vi "Test DIO.vi"() -> ()   [LabVIEW 2012]
uses:
  <vilib>/DAQmx/write.llb/DAQmx Write (Digital 2D Bool NChan 1Samp NLine).vi
  <vilib>/DAQmx/read.llb/DAQmx Read (Digital 2D Bool NChan 1Samp NLine).vi
  <vilib>/DAQmx/create/channels.llb/DAQmx Create Channel (DO-Digital Output).vi
  <vilib>/DAQmx/miscellaneous.llb/DAQmx Fill In Error Info.vi
panel:
  out "data read":bool[][](array[boolean])
  in  "data":bool[][](array[boolean])
  out "number of samples written per channel":u32
  in  "stop":bool
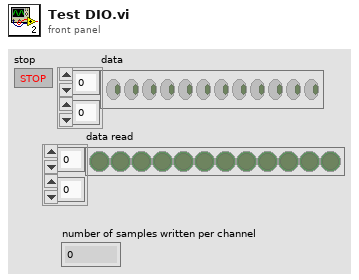
[diagram p1: front panel]
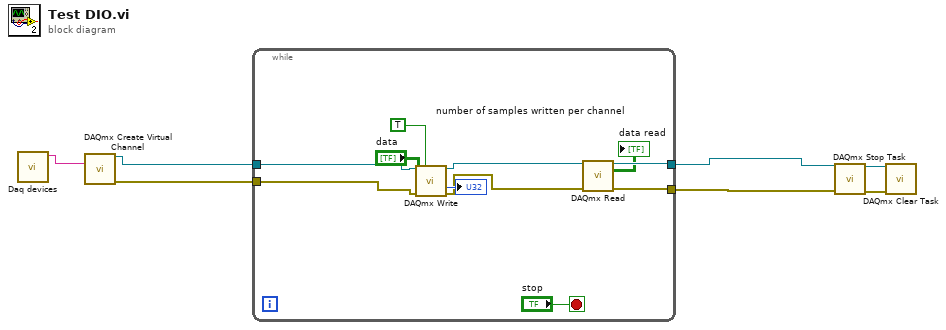
[diagram p0: block diagram]
diagram:
  n1 = call "Daq devices.vi"() -> ("DO"=w1:string)  [unwired: 6 in, 4 out]
  n2 = call-poly <vilib>:"DAQmx Create Virtual Channel.vi"("lines"=w1) -> ("task out"=w7:refnum<k21>, "error out"=w6:errorcluster)  [unwired: 13 in]
  n3 = while {
    tunnel: w7 -> [w16]
    tunnel: w6 -> [w17]
    tunnel: [w11] -> w2
    tunnel: [w9] -> w3
    stop <- "stop" stop-if-true
    n4 = call-poly <vilib>:"DAQmx Write.vi"("task/channels in"=w16, "auto start"=TRUE, "data"="data", "error in"=w17) -> ("task out"=w12:refnum<k21>, "number of samples written per channel"=→"number of samples written per channel":u32, "error out"=w10:errorcluster)  [unwired: 9 in]
    n5 = call-poly <vilib>:"DAQmx Read.vi"("task/channels in"=w12, "error in"=w10) -> ("task out"=w11:refnum<k21>, "data"=→"data read":bool[][], "error out"=w9:errorcluster)  [unwired: 11 in]
  }
  n6 = call <vilib>:"DAQmx Stop Task.vi"("task/channels in"=w2, "error in"=w3) -> ("task out"=w5:refnum<k21>, "error out"=w4:errorcluster)  [unwired: 12 in]
  n7 = call <vilib>:"DAQmx Clear Task.vi"("task in"=w5, "error in"=w4) -> ()  [unwired: 13 in, 1 out]
